vi "save control values.vi"(5 "Append timestamp (true)":bool=TRUE, 6 "error in":errorcluster, 8 "Dont save":string[](array[string]), 9 "Path":path) -> (0 "error out":errorcluster, 3 "file path out":path)   [LabVIEW 2009, in "POLARIS Vision utility.lvlib"]
doc: "from ni.com \nauthor mmiers."
uses:
  POLARIS Vision utility.lvlib
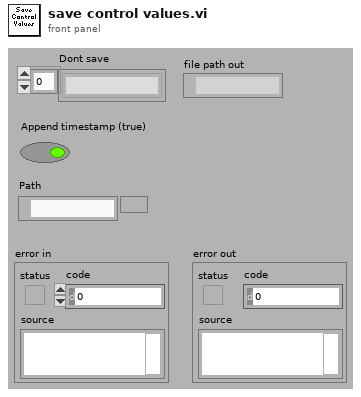
[diagram p1: front panel]
types:
  T1 = cluster{"Name":string, "type string":i16[], "data string":string}[]
  T2 = enum32{"invalid app kind", "Development System", "Run Time System", "Student Edition", "Embedded LabVIEW", "Evaluation", "Custom"}
  T3 = cluster{"Name":string, "type string":i16[], "data string":string}
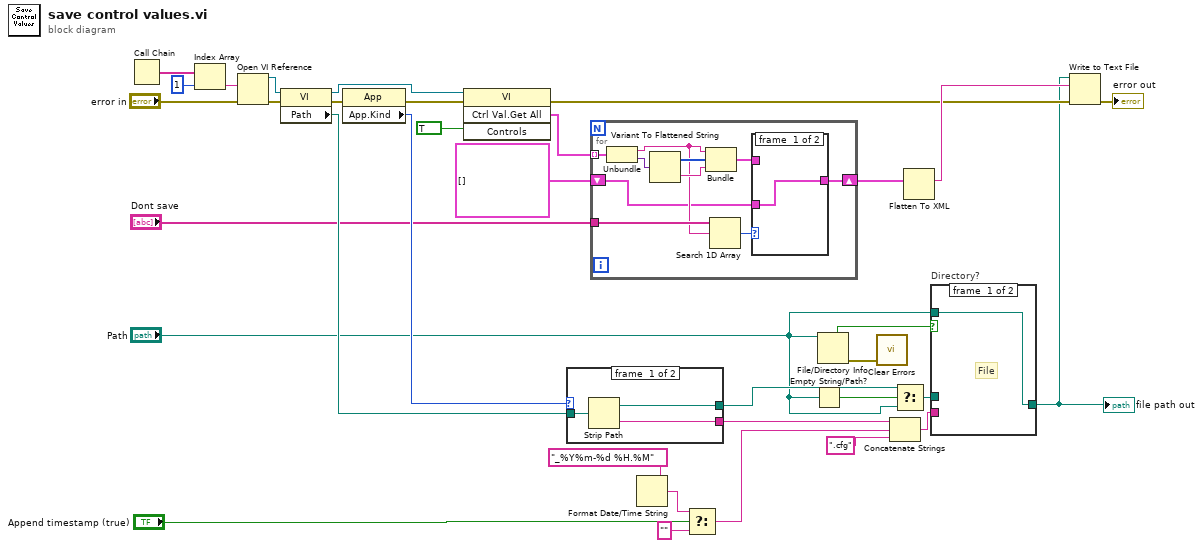
[diagram p0: block diagram]
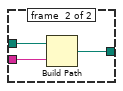
[diagram p2: hidden frame]
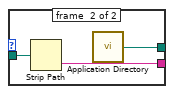
[diagram p3: hidden frame]
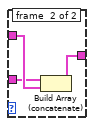
[diagram p4: hidden frame]
diagram:
  n1 = Call Chain() -> (call chain=w29:string[])
  n2 = Index Array(array=w29, index=1) -> (element=w25:string)
  n3 = Open VI Reference(vi path=w25, error in (no error)="error in") -> (vi reference=w24:refnum<vi>, error out=w26:errorcluster)  [unwired: 4 in]
  n4 = property class="VI"(reference=w24, error in=w26) -> (reference out=w4:refnum<vi>, error out=w21:errorcluster, "Path"=w23:path)
  n5 = property class="App"(error in=w21) -> (error out=w20:errorcluster, "App.Kind"=w22:T2)  [unwired: 1 in, 1 out]
  n6 = invoke class="VI" method="Ctrl Val.Get All"(reference=w4, error in=w20, "Controls"=TRUE ("Save control values")) -> (error out=w31:errorcluster, "Get All Control Values Variant"=w2:cluster{"Name":string, "Variant Data":variant}[])  [unwired: 1 in, 2 out]
  n7 = case shown="\"Run Time System\"" w22 {
    tunnel: w23 -> [w37 w40]
    tunnel: [w36 w39] -> w10
    tunnel: [w35 w38] -> w15
    frame #0 {
      n8 = Strip Path(path=w37) -> (stripped path=w36:path, name=w35:string)
    }
    frame #1 {
      n9 = Strip Path(path=w40) -> (name=w38:string)  [unwired: 1 out]
      n10 = call <vilib>:"Application Directory.vi"() -> ("Application Directory"=w39:path)
    }
  }
  n11 = for {
    tunnel: w2 -> [w47] mode=indexing
    tunnel: "Dont save" -> [w46]
    shift-right: [w42] -> w32
    shift-left: T1 [] -> [w41]
    n12 = Unbundle(w47) -> ("Name"=w45:string, "Variant Data"=w50:variant)
    n13 = Variant To Flattened String(Variant=w50) -> (data string=w48:string, 1:w49:i16[])
    n14 = Bundle("Name"=w45, "type string"=w49, "data string"=w48) -> (w43:T3)  [unwired: 1 out]
    n15 = Search 1D Array(1D array=w46, element=w45) -> (index of element=w44:i32)  [unwired: 1 in]
    n16 = case shown="0, Default" w44 {
      tunnel: w43 -> [_ w54]
      tunnel: [w51 w53] -> w42
      tunnel: w41 -> [w51 w52]
      frame #0 {
      }
      frame #1 {
        n17 = Build Array (concatenate)(w52, w54) -> (w53:T1)
      }
    }
  }
  n18 = Format Date/Time String(time format string (%c)="_%Y%m-%d %H.%M") -> (date/time string=w13:string)  [unwired: 2 in]
  n19 = Select(t=w13, s="Append timestamp (true)", f="") -> (s? t:f=w12:string)
  n20 = Empty String/Path?(string/path="Path") -> (empty?=w9:bool)
  n21 = File/Directory Info(path="Path") -> (directory=w7:bool, error out=w5:errorcluster)  [unwired: 1 in, 5 out]
  n22 = call <vilib>:"Clear Errors.vi"("error in (no error)"=w5) -> ()  [unwired: 6 in, 1 out]
  n23 = Concatenate Strings(w15, w12, ".cfg" ("string")) -> (w18:string)
  n24 = Select(t=w10, s=w9, f="Path") -> (s? t:f=w8:path)
  n25 = Flatten To XML(anything=w32) -> (xml string=w33:string)
  n26 = case "Directory?" shown="True" w7 {
    tunnel: [w55 w58] -> w19
    tunnel: w18 -> [_ w57]
    tunnel: w8 -> [_ w56]
    tunnel: "Path" -> [w55 _]
    frame #0 {
      # "File"
    }
    frame #1 {
      n27 = Build Path(base path=w56, name or relative path=w57) -> (appended path=w58:path)
    }
  }
  "file path out" <- w19
  n28 = Write to Text File(file (use dialog)=w19, text=w33, error in=w31) -> (error out=→"error out":errorcluster)  [unwired: 3 out]
